vi "FliePackageTransfer.vi"(6 "TransferMode":T1, 8 "error in":errorcluster caption="错误输入（无错误）", 10 "TbcFilePath":string="C:\\Users\\Administrator\\Desktop\\Xmodem_2\\test.txt", 11 "ComIn":refnum<visa-resource-name>="COM16") -> (0 "error out":errorcluster caption="错误输出", 1 "MD5":string, 2 "FeedBack":string[](array[string]), 3 "Result":bool)   [LabVIEW 2013]
uses:
  TransferMode.ctl
  <vilib>/Instr/_visa.llb/VISA Flush IO Buffer Mask.ctl
  <vilib>/Instr/_visa.llb/VISA Configure Serial Port (Instr).vi
  Global.vi
panel:
  out "读取缓冲区":string
  out "x/y":dbl
  out "反转":string
  out "长度2":i32
  out "trimmedstring":string caption="删减后字符串"
  out "字符串":string
  out "SinglePacket":string
  out "接收显示":string
  out "数组 2":i32[](array[numeric])
  out "数组":string[](array[string])
  out "长度":i32
  out "DataPack":string[](array[string])
  out "数值":i32
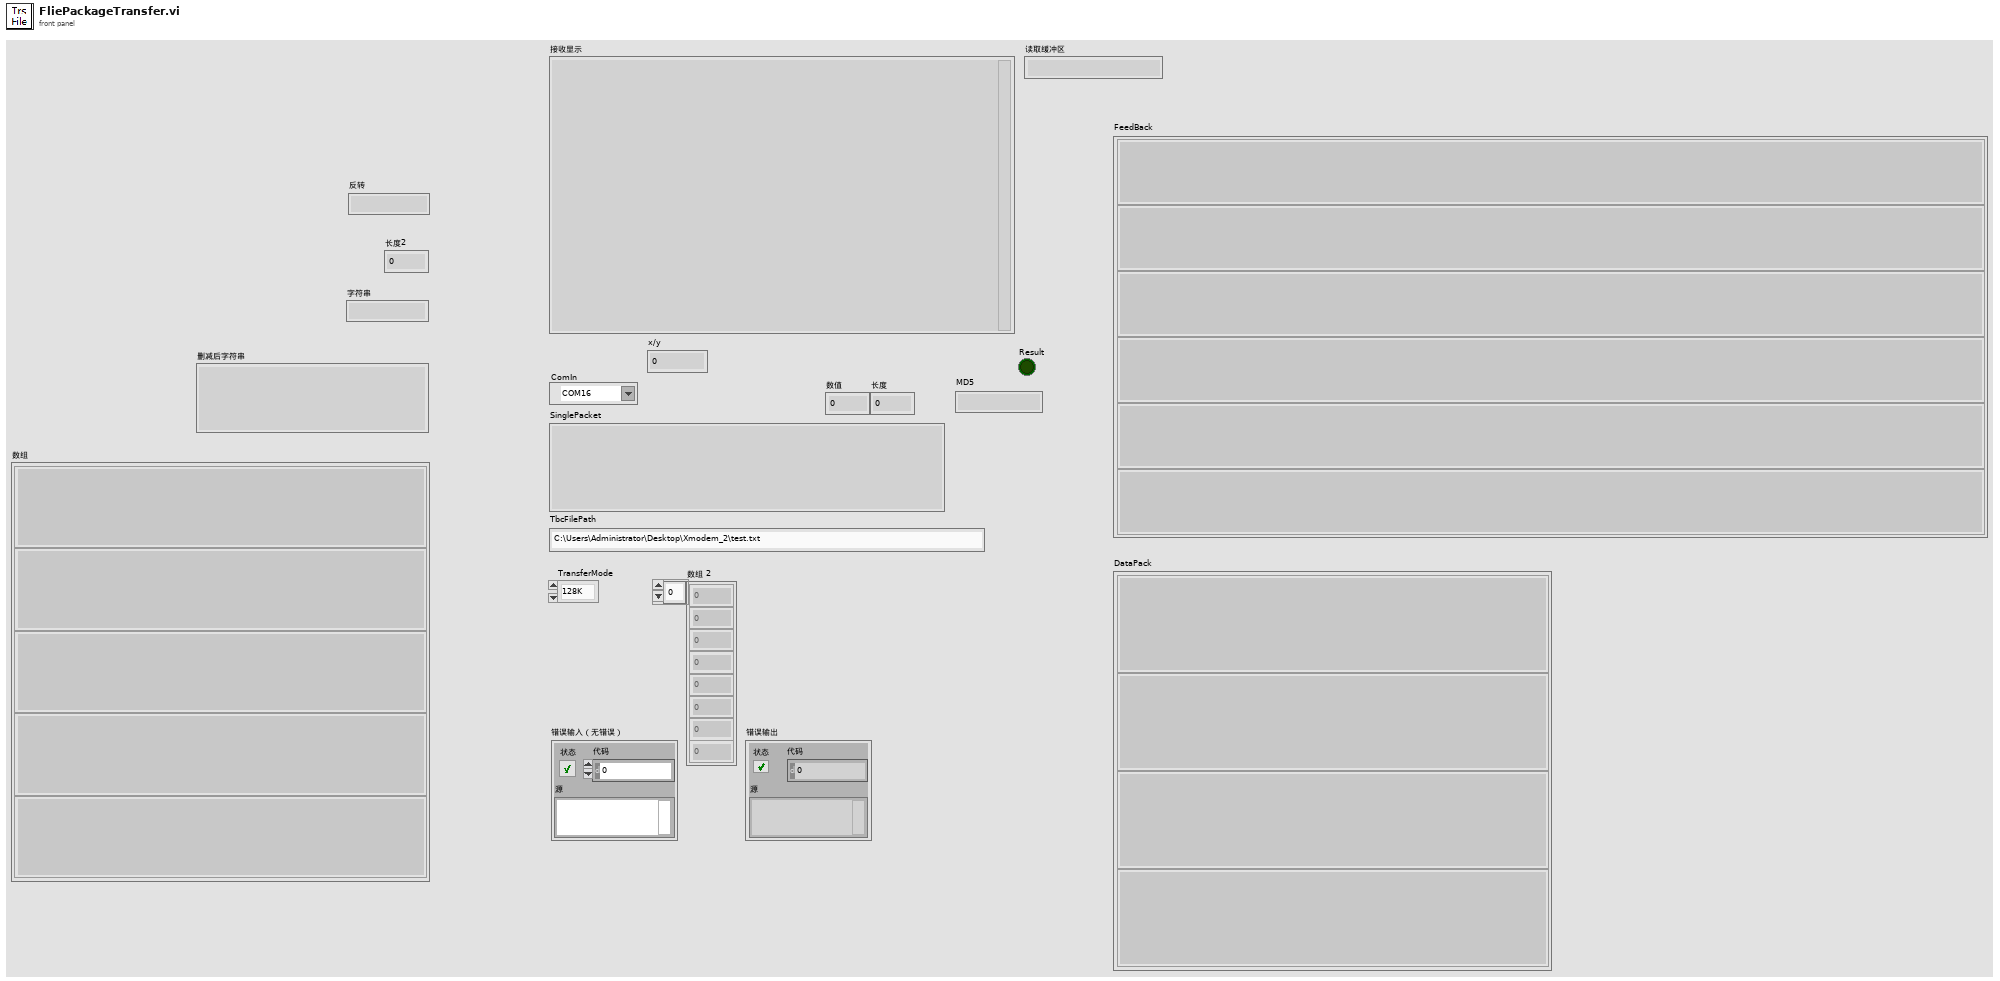
[diagram p1: front panel]
types:
  T1 = typedef "TransferMode.ctl" = enum16{"128K", "1024K"}
  T2 = typedef "VISA Flush IO Buffer Mask.ctl" = u16
  T3 = cluster{"波特率":u32, "数据比特":u16, "奇偶":enum16{"None", "Odd", "Even", "Mark", "Space"}, "停止位":u16, "流控制":u16}
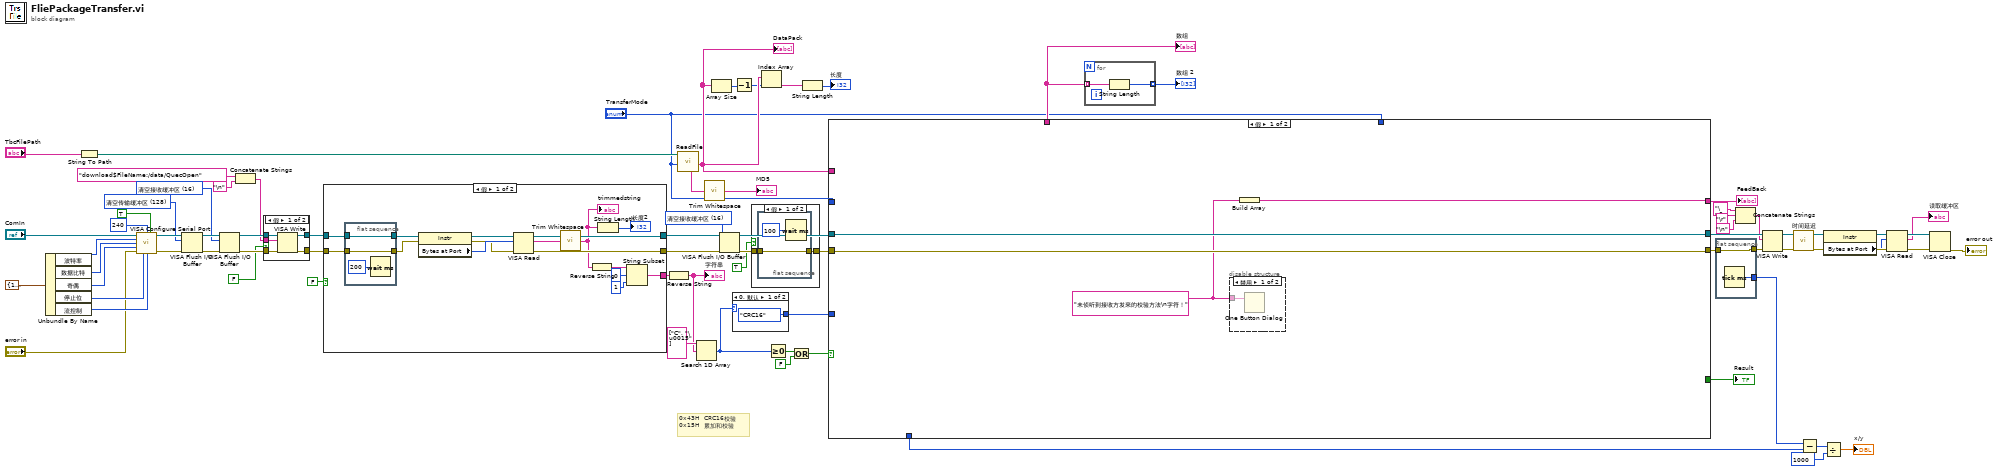
[diagram p0: block diagram]
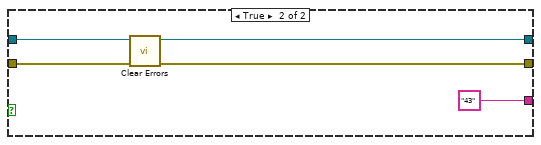
[diagram p4: hidden frame]
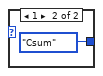
[diagram p5: hidden frame]
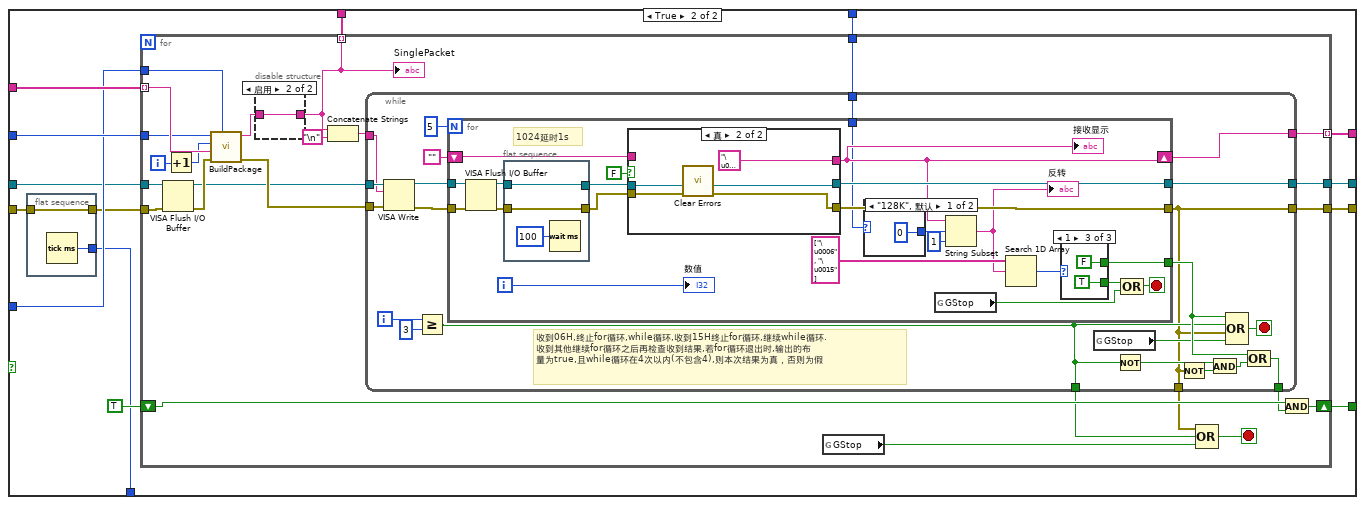
[diagram p7: hidden frame]
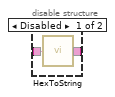
[diagram p8: hidden frame]
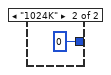
[diagram p9: hidden frame]
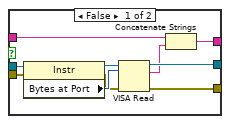
[diagram p10: hidden frame]
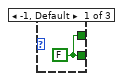
[diagram p11: hidden frame]
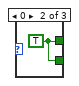
[diagram p12: hidden frame]
diagram:
  w24 = T2 16 items=["清空接收缓冲区"=16, "向设备写入传输缓冲区"=32, "清空接收缓冲区（无I/O）"=64, "清空传输缓冲区"=128] ("Mask")
  w60 = T2 16 items=["清空接收缓冲区"=16, "向设备写入传输缓冲区"=32, "清空接收缓冲区（无I/O）"=64, "清空传输缓冲区"=128] ("Mask")
  w63 = T2 128 items=["清空接收缓冲区"=16, "向设备写入传输缓冲区"=32, "清空接收缓冲区（无I/O）"=64, "清空传输缓冲区"=128] ("Mask")
  # "0x43H  CRC16校验\n0x15H  累加和校验"
  n1 = Unbundle By Name(T3 {"波特率"=115200, "数据比特"=8, "奇偶"=enum."None", "停止位"=10, "流控制"=0} ("串口设置")) -> ("波特率"=w72:u32, "数据比特"=w71:u16, "奇偶"=w70:enum16{"None", "Odd", "Even", "Mark", "Space"}, "停止位"=w69:u16, "流控制"=w68:u16)
  n2 = String To Path(string="TbcFilePath") -> (path=w57:path)
  n3 = call-poly "VISA Configure Serial Port"("VISA resource name"="ComIn", "termination char\n(0xA = '\\n' = LF)"=u8 240 ("termination char\n(0xA = '\\n' = LF)"), "Enable Termination\nChar (T)"=TRUE ("Enable Termination\nChar (T)"), "baud rate (9600)"=w72, "data bits (8)"=w71, "parity (0:none)"=w70, "error in (no error)"="error in", "stop bits (10: 1 bit)"=w69, "flow control (0:none)"=w68) -> ("VISA resource name out"=w65:refnum<visa-resource-name>, "error out"=w64:errorcluster)  [unwired: 5 in]
  n4 = VISA Flush I/O Buffer(VISA resource name=w65, mask (16)=w63, error in (no error)=w64) -> (VISA resource name out=w61:refnum<visa-resource-name>, error out=w62:errorcluster)
  n5 = VISA Flush I/O Buffer(VISA resource name=w61, mask (16)=w60, error in (no error)=w62) -> (VISA resource name out=w44:refnum<visa-resource-name>, error out=w28:errorcluster)
  n6 = Concatenate Strings("download$FileName:/data/QuecOpen", "\n") -> (w42:string)
  n7 = case shown="假" FALSE {
    tunnel: w44 -> [w79 w81]
    tunnel: w42 -> [w78 _]
    tunnel: [w77 w81] -> w34
    tunnel: [w76 w80] -> w29
    tunnel: w28 -> [w75 w80]
    frame False {
      n8 = VISA Write(VISA resource name=w79, write buffer=w78, error in (no error)=w75) -> (VISA resource name out=w77:refnum<visa-resource-name>, error out=w76:errorcluster)  [unwired: 1 out]
    }
    frame True {
    }
  }
  n9 = case shown="假" FALSE {
    tunnel: w29 -> [w97 w103]
    tunnel: [w96 w101] -> w23
    tunnel: [w95 w104] -> w56
    tunnel: [w94 "43"] -> w45
    tunnel: w34 -> [w93 w104]
    frame False {
      n10 = flat-sequence {
        tunnel: w97 -> [w100]
        tunnel: [w100] -> w85
        tunnel: [w98] -> w84
        tunnel: w93 -> [w98]
        frame #0 {
          n11 = Wait (ms)(milliseconds to wait=u32 200 ("等待时间（毫秒）")) -> ()  [unwired: 1 out]
        }
      }
      n12 = property class="Instr"(reference=w84, error in=w85) -> (reference out=w89:refnum<visa-resource-name>, error out=w87:errorcluster, "Bytes at Port"=w88:u32)
      n13 = VISA Read(VISA resource name=w89, byte count=w88, error in (no error)=w87) -> (VISA resource name out=w95:refnum<visa-resource-name>, read buffer=w86:string, error out=w96:errorcluster)  [unwired: 1 out]
      n14 = call <vilib>:"Trim Whitespace.vi"("string"=w86) -> ("trimmed string"=w83:string)  [unwired: 1 in]
      "trimmedstring" <- w83
      n15 = Reverse String(1:w83) -> (0:w92:string)
      n16 = String Length(string=w83) -> (length=→"长度2":i32)
      n17 = String Subset(string=w92, offset (0)=0 ("偏移量(0)"), length (rest)=1 ("偏移量(0)")) -> (substring=w94:string)
    }
    frame True {
      n18 = call <vilib>:"Clear Errors.vi"("error in (no error)"=w103) -> ("error out"=w101:errorcluster)  [unwired: 6 in]
    }
  }
  n19 = Reverse String(1:w45) -> (0:w26:string)
  "字符串" <- w26
  n20 = call "ReadFile.vi"("TransferMode"="TransferMode", "FilePath"=w57) -> ("DataPack"=w39:string[], "MD5"=w2:string)  [unwired: 4 in, 4 out]
  "DataPack" <- w39
  n21 = Search 1D Array(1D array=string[] ["C", "\u0015"], element=w26) -> (index of element=w55:i32)  [unwired: 1 in]
  n22 = call <vilib>:"Trim Whitespace.vi"("string"=w2) -> ("trimmed string"=→"MD5":string)  [unwired: 1 in]
  n23 = Array Size(array=w39) -> (size(s)=w37:i32)
  n24 = VISA Flush I/O Buffer(VISA resource name=w56, mask (16)=w24, error in (no error)=w23) -> (VISA resource name out=w25:refnum<visa-resource-name>, error out=w22:errorcluster)
  n25 = case shown="0, 默认" w55 {
    tunnel: [enum16{"Csum", "CRC16"}."CRC16" ("ErrorCheck") enum16{"Csum", "CRC16"}."Csum" ("ErrorCheck")] -> w54
    frame 0, Default {
    }
    frame 1 {
    }
  }
  n26 = Decrement(x=w37) -> (x-1=w38:i32)
  n27 = case shown="假" TRUE {
    tunnel: w22 -> [w108 w111]
    tunnel: [w107 w111] -> w21
    frame False {
      n28 = flat-sequence {
        tunnel: w108 -> [w109]
        tunnel: [w109] -> w107
        frame #0 {
          n29 = Wait (ms)(milliseconds to wait=u32 100 ("等待时间（毫秒）")) -> ()  [unwired: 1 out]
        }
      }
    }
    frame True {
    }
  }
  n30 = Index Array(array=w39, index=w38) -> (element=w41:string)
  n31 = Greater Or Equal To 0?(x=w55) -> (x >= 0?=w32:bool)
  n32 = Or(x=w32, y=FALSE) -> (x .or. y?=w31:bool)
  n33 = String Length(string=w41) -> (length=→"长度":i32)
  n34 = case shown="假" w31 {
    tunnel: w21 -> [w114 w118]
    tunnel: w25 -> [w115 w127]
    tunnel: w39 -> [_ w130]
    tunnel: "TransferMode" -> [_ w129]
    tunnel: w54 -> [_ w128]
    tunnel: [w115 w126] -> w53
    tunnel: [w114 w125] -> w14
    tunnel: [w112 w124] -> w52
    tunnel: [_ w122] -> w51
    tunnel: [_ w121] -> w36
    tunnel: "TransferMode" -> [_ w120]
    tunnel: [_ w117] -> w12
    frame False {
      w113 = "未侦听到接收方发来的校验方法\n字符！" ("消息")
      n35 = disable-structure shown="禁用" {
        disable-tunnel: w113 -> [w116 _]
        frame Disabled {
          n36 = One Button Dialog(message=w116) -> ()  [unwired: 1 in, 1 out]
        }
        frame Enabled {
        }
      }
      n37 = Build Array(w113) -> (w112:string[])
    }
    frame True {
      n38 = flat-sequence {
        tunnel: [w132] -> w119
        tunnel: w118 -> [w132]
        tunnel: [w131] -> w117
        frame #0 {
          n39 = Tick Count (ms)() -> (millisecond timer value=w131:u32)
        }
      }
      n40 = for {
        tunnel: w130 -> [w157] mode=indexing
        tunnel: w129 -> [w154]
        tunnel: w128 -> [w153]
        tunnel: w127 -> [w151]
        tunnel: w119 -> [w149]
        tunnel: [w147] -> w126
        tunnel: [w146] -> w125
        tunnel: [w145] -> w124 mode=indexing
        shift-right: [w144] -> w122
        shift-left: TRUE -> [w143]
        tunnel: [w136] -> w121 mode=indexing
        tunnel: w120 -> [w133]
        i -> [w156]
        stop <- w141 stop-if-true
        n41 = VISA Flush I/O Buffer(VISA resource name=w151, error in (no error)=w149) -> (VISA resource name out=w148:refnum<visa-resource-name>, error out=w150:errorcluster)  [unwired: 1 in]
        n42 = Increment(x=w156) -> (x+1=w155:i32)
        n43 = call "BuildPackage.vi"("ErrorCheck"=w153, "error in"=w150, "DataBytes"=w157, "sequence"=w155, "TransferMode"=w154) -> ("error out"=w152:errorcluster, "Packet"=w137:string)  [unwired: 5 in]
        n44 = disable-structure shown="启用" {
          disable-tunnel: w137 -> [w159 w160]
          disable-tunnel: [w158 w160] -> w136
          frame Disabled {
            n45 = call "HexToString.vi"("StrIn"=w159) -> ("StrOut"=w158:string)
          }
          frame Enabled {
          }
        }
        "SinglePacket" <- w136
        n46 = Concatenate Strings(w136, "\n") -> (w134:string)
        n47 = while {
          tunnel: w148 -> [w181]
          tunnel: w152 -> [w180]
          tunnel: w134 -> [w179]
          tunnel: [w176] -> w147
          tunnel: [w162] -> w146
          tunnel: [w171] -> w145
          tunnel: [w168] -> w142
          tunnel: [w166] -> w140
          tunnel: [w162] -> w138
          tunnel: w133 -> [w161]
          i -> [w175]
          stop <- w173 stop-if-true
          # "收到06H,终止for循环,while循环,收到15H终止for循环,继续while循环.\n收到其他继续for循环之后再检查收到结果,若for循环退出时,输出的布\n量为true,且while循环在4次以内(不包含4),则本次结果为真，否则为假"
          n48 = VISA Write(VISA resource name=w181, write buffer=w179, error in (no error)=w180) -> (VISA resource name out=w178:refnum<visa-resource-name>, error out=w177:errorcluster)  [unwired: 1 out]
          n49 = Greater Or Equal?(x=w175, y=3) -> (x >= y?=w166:bool)
          n50 = for {
            N: 5 -> [_]
            tunnel: w178 -> [w202]
            tunnel: w177 -> [w201]
            tunnel: [w199] -> w176
            tunnel: [w198] -> w162
            shift-right: [w184] -> w171
            shift-left: "" -> [w197]
            tunnel: [w194] -> w169
            tunnel: w161 -> [w182]
            i -> [w190]
            stop <- w193 stop-if-true
            # "1024延时1s"
            n51 = VISA Flush I/O Buffer(VISA resource name=w202) -> (VISA resource name out=w187:refnum<visa-resource-name>)  [unwired: 2 in, 1 out]
            n52 = flat-sequence {
              tunnel: w187 -> [w224]
              tunnel: w201 -> [w223]
              tunnel: [w224] -> w188
              tunnel: [w223] -> w200
              frame #0 {
                n53 = Wait (ms)(milliseconds to wait=u32 100 ("等待时间（毫秒）")) -> ()  [unwired: 1 out]
              }
            }
            n54 = case shown="真" FALSE {
              tunnel: w200 -> [w214 w217]
              tunnel: [w213 w215] -> w199
              tunnel: [w212 w216] -> w198
              tunnel: w197 -> [w211 _]
              tunnel: [w206 "\u0006"] -> w184
              tunnel: w188 -> [w205 w215]
              frame False {
                n55 = property class="Instr"(reference=w205, error in=w214) -> (reference out=w210:refnum<visa-resource-name>, error out=w208:errorcluster, "Bytes at Port"=w209:u32)
                n56 = VISA Read(VISA resource name=w210, byte count=w209, error in (no error)=w208) -> (VISA resource name out=w213:refnum<visa-resource-name>, read buffer=w207:string, error out=w212:errorcluster)  [unwired: 1 out]
                n57 = Concatenate Strings(w211, w207) -> (w206:string)
              }
              frame True {
                n58 = call <vilib>:"Clear Errors.vi"("error in (no error)"=w217) -> ("error out"=w216:errorcluster)  [unwired: 6 in]
              }
            }
            "接收显示" <- w184
            n59 = case shown="\"128K\", 默认" w182 {
              tunnel: [0 ("偏移量(0)") 0 ("偏移量(0)")] -> w185
              frame "128K", Default {
              }
              frame "1024K" {
              }
            }
            n60 = global read "Global.vi" "GStop"() -> (w191:bool)
            n61 = String Subset(string=w184, offset (0)=w185, length (rest)=1 ("长度（剩余）")) -> (substring=w183:string)
            "反转" <- w183
            n62 = Search 1D Array(1D array=string[] ["\u0006", "\u0015"], element=w183) -> (index of element=w195:i32)  [unwired: 1 in]
            n63 = case shown="1" w195 {
              tunnel: [w219 w220 TRUE] -> w192
              tunnel: [w219 w220 FALSE] -> w194
              frame -1, Default {
                w219 = FALSE
              }
              frame 0 {
                w220 = TRUE
              }
              frame 1 {
              }
            }
            n64 = Compound Arithmetic op=OR(w192, w191) -> (w193:bool)
            "数值" <- w190
          }
          n65 = global read "Global.vi" "GStop"() -> (w167:bool)
          n66 = Not(x=w166) -> (.not. x?=w165:bool)
          n67 = Not(x=w162) -> (.not. x?=w163:bool)
          n68 = And(x=w165, y=w163) -> (x .and. y?=w164:bool)
          n69 = Compound Arithmetic op=OR(w169, w166, w162, w167) -> (w173:bool)
          n70 = Compound Arithmetic op=OR(w169, w164) -> (w168:bool)
        }
        n71 = global read "Global.vi" "GStop"() -> (w139:bool)
        n72 = Compound Arithmetic op=OR(w138, w140, w139) -> (w141:bool)
        n73 = And(x=w143, y=w142) -> (x .and. y?=w144:bool)
      }
    }
  }
  "FeedBack" <- w52
  "Result" <- w51
  "数组" <- w36
  n74 = for {
    tunnel: w36 -> [w227] mode=indexing
    tunnel: [w226] -> w35 mode=indexing
    n75 = String Length(string=w227) -> (length=w226:i32)
  }
  "数组 2" <- w35
  n76 = flat-sequence {
    tunnel: [w229] -> w15
    tunnel: w14 -> [w229]
    tunnel: [w228] -> w13
    frame #0 {
      n77 = Tick Count (ms)() -> (millisecond timer value=w228:u32)
    }
  }
  n78 = Concatenate Strings("\u0004", "\r", "\n") -> (w17:string)
  n79 = VISA Write(VISA resource name=w53, write buffer=w17, error in (no error)=w15) -> (VISA resource name out=w50:refnum<visa-resource-name>, error out=w48:errorcluster)  [unwired: 1 out]
  n80 = call "时间延迟"("error in (no error)"=w48) -> ("error out"=w47:errorcluster)  [unwired: 10 in]
  n81 = Subtract(x=w13, y=w12) -> (x-y=w11:u32)
  n82 = property class="Instr"(reference=w50) -> (reference out=w8:refnum<visa-resource-name>, "Bytes at Port"=w6:u32)  [unwired: 1 in, 1 out]
  n83 = Divide(x=w11, y=1000) -> (x/y=→"x/y":dbl)
  n84 = VISA Read(VISA resource name=w8, byte count=w6) -> (VISA resource name out=w7:refnum<visa-resource-name>, read buffer=→"读取缓冲区":string)  [unwired: 1 in, 2 out]
  n85 = VISA Close(VISA resource name=w7, error in (no error)=w47) -> (error out=→"error out":errorcluster)
